vi "Remove Quotes.vi"(8 "error in (no error)":errorcluster, 11 "string":string) -> (0 "error out":errorcluster, 1 "in quotes?":bool, 3 "without quotes":string)   [LabVIEW 2010, in "NI_LVConfig.lvlib"]
uses:
  NI_LVConfig.lvlib
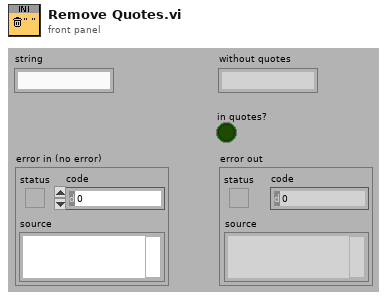
[diagram p1: front panel]
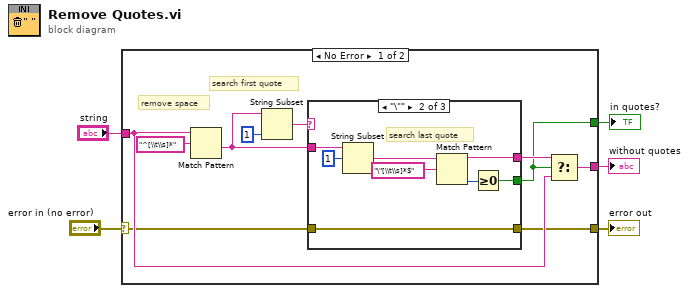
[diagram p0: block diagram]
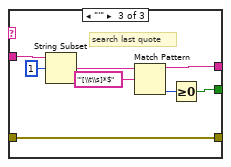
[diagram p3: hidden frame]
diagram:
  n1 = case shown="No Error" "error in (no error)" {
    selector: "error in (no error)" -> [w6 w34]
    tunnel: [w9 w33] -> w5
    tunnel: "string" -> [w10 w33]
    tunnel: [w7 w34] -> w3
    tunnel: [w8 _] -> w2
    frame No Error {
      # "remove space"
      # "search first quote"
      n2 = Match Pattern(string=w10, regular expression="^[\\t\\s]*") -> (after substring=w15:string)  [unwired: 1 in, 3 out]
      n3 = String Subset(string=w15, length (rest)=1 ("length (rest)")) -> (substring=w13:string)  [unwired: 1 in]
      n4 = case shown="\"\\\"\"" w13 {
        tunnel: [_ w23 w30] -> w8
        tunnel: [_ w22 w31] -> w14
        tunnel: w15 -> [_ w20 w28]
        tunnel: w6 -> [w16 w18 w26]
        tunnel: [w16 w18 w26] -> w7
        frame Default {
        }
        frame "\"" {
          # "search last quote"
          n5 = String Subset(string=w20, offset (0)=1 ("length (rest)")) -> (substring=w19:string)  [unwired: 1 in]
          n6 = Match Pattern(string=w19, regular expression="\"[\\t\\s]*$") -> (before substring=w22:string, offset past match=w17:i32)  [unwired: 1 in, 2 out]
          n7 = Greater Or Equal To 0?(x=w17) -> (x >= 0?=w23:bool)
        }
        frame "'" {
          # "search last quote"
          n8 = String Subset(string=w28, offset (0)=1 ("length (rest)")) -> (substring=w27:string)  [unwired: 1 in]
          n9 = Match Pattern(string=w27, regular expression="'[\\t\\s]*$") -> (before substring=w31:string, offset past match=w25:i32)  [unwired: 1 in, 2 out]
          n10 = Greater Or Equal To 0?(x=w25) -> (x >= 0?=w30:bool)
        }
      }
      n11 = Select(t=w14, s=w8, f=w10) -> (s? t:f=w9:string)
    }
    frame Error {
    }
  }
  "without quotes" <- w5
  "error out" <- w3
  "in quotes?" <- w2
